vi "TimeStmp2DB (Date).vi"(11 "Login info (start)":timestamp) -> (3 "result string":string)   [LabVIEW 2019]
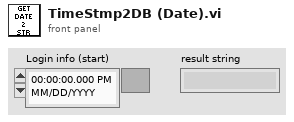
[diagram p1: front panel]
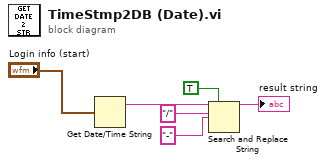
[diagram p0: block diagram]
diagram:
  n1 = Get Date/Time String(seconds (now)="Login info (start)") -> (date string=w1:string)  [unwired: 2 in, 1 out]
  n2 = Search and Replace String(replace all?=TRUE ("replace all? (F)"), input string=w1, search string="/" ("replace string (\"\")"), replace string="-" ("replace string (\"\")")) -> (result string=→"result string":string)  [unwired: 4 in, 3 out]
